vi "Init Control Captions.vi"(8 "error in (no error)":errorcluster, 11 "Custom Data Cluster In":T1) -> (0 "error out":errorcluster, 3 "Custom Data Cluster Out":T1)   [LabVIEW 2011]
doc: "This VI will put the full path back into the Caption for each control"
uses:
  Custom Data Cluster Control.ctl
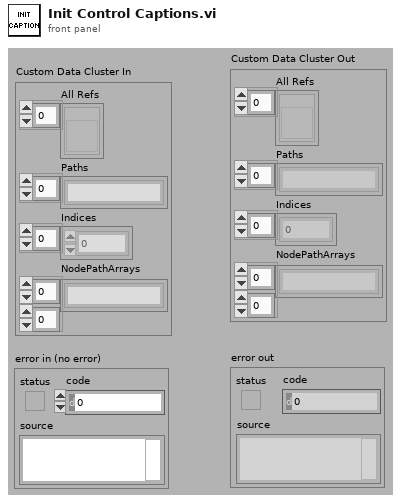
[diagram p1: front panel]
types:
  T1 = typedef "Custom Data Cluster Control.ctl" = cluster{"All Refs":refnum<vi>[], "Paths":string[], "Indices":u32[], "NodePathArrays":string[][]}
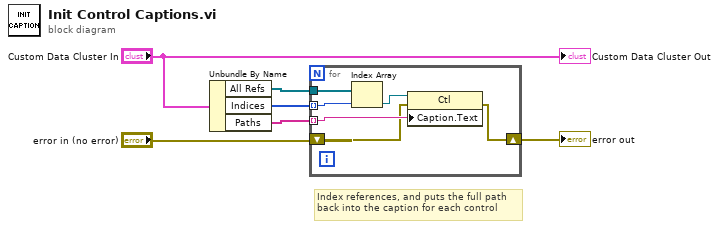
[diagram p0: block diagram]
diagram:
  # "Index references, and puts the full path\nback into the caption for each control"
  n1 = Unbundle By Name("Custom Data Cluster In") -> ("All Refs"=w6:refnum<vi>[], "Indices"=w5:u32[], "Paths"=w4:string[])
  n2 = for {
    tunnel: w6 -> [w11]
    tunnel: w5 -> [w12] mode=indexing
    tunnel: w4 -> [w9] mode=indexing
    shift-right: [w7] -> w1
    shift-left: "error in (no error)" -> [w8]
    n3 = Index Array(array=w11, index=w12) -> (element=w10:refnum<vi>)
    n4 = property class="Ctl"(reference=w10, error in=w8, "Caption.Text"=w9) -> (error out=w7:errorcluster)  [unwired: 1 out]
  }
  "error out" <- w1
  "Custom Data Cluster Out" <- "Custom Data Cluster In"
